vi "Read Output.vi"(8 "error in":errorcluster, 10 "byte count":i32=1000, 11 "GOLPI ref. in":T1={"pipe handle"={"lv_proc.dll file path"=path "", "process instance handle"=[]}, "fast read timeout [ms]"=500, "fast read settle time [ms]"=10, "fast read to multiple [ms]"=1, "max elements per input line"=100, "slow read timeout [ms]"=5000, "stdin double format specifier"="%_16e", "max elements per stdout output column"=100}) -> (0 "error out":errorcluster, 2 "read buffer":string, 3 "GOLPI ref. out":T1={"pipe handle"={"lv_proc.dll file path"=path "", "process instance handle"=[]}, "fast read timeout [ms]"=500, "fast read settle time [ms]"=10, "fast read to multiple [ms]"=1, "max elements per input line"=100, "slow read timeout [ms]"=5000, "stdin double format specifier"="%_16e", "max elements per stdout output column"=100}, 5 "bytes remaining":i32)   [LabVIEW 2013, in "GOLPI library.lvlib"]
doc: "Reads output of GNU Octave buffered in stdout pipe. Returns number of bytes remaining in the stdout (if any)."
uses:
  GOLPI library.lvlib
  Private/Type Definitions/GOLPI reference Type Def.ctl
  LV Process source distribution/Pipe Handle.ctl
  LV Process source distribution/LV Process library.lvlib
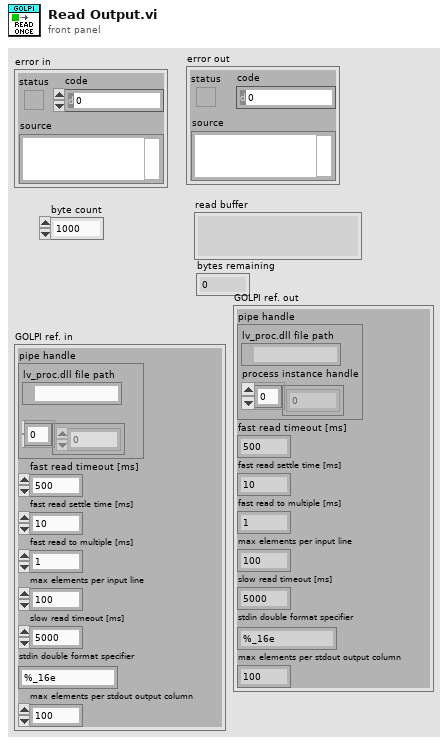
[diagram p1: front panel]
types:
  T1 = typedef "GOLPI library.lvlib/GOLPI reference Type Def.ctl" = cluster{"pipe handle":T2, "fast read timeout [ms]":u32, "fast read settle time [ms]":u32, "fast read to multiple [ms]":u32, "max elements per input line":u32, "slow read timeout [ms]":u32, "stdin double format specifier":string, "max elements per stdout output column":u32}
  T2 = typedef "LV Process library.lvlib/Pipe Handle.ctl" = cluster{"lv_proc.dll file path":path, "process instance handle":u32[]}
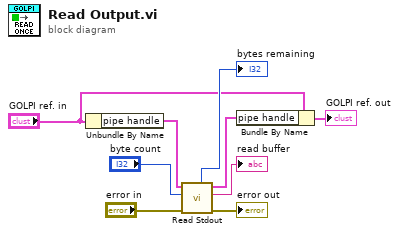
[diagram p0: block diagram]
diagram:
  n1 = Unbundle By Name("GOLPI ref. in") -> ("pipe handle"=w2:T2)
  n2 = call "Read Stdout.vi"("error in"="error in", "byte count"="byte count", "pipe in"=w2) -> ("error out"=→"error out":errorcluster, "read buffer"=→"read buffer":string, "pipe out"=w1:T2, "bytes remaining"=→"bytes remaining":i32)  [unwired: 3 in, 2 out]
  n3 = Bundle By Name(cluster="GOLPI ref. in", "pipe handle"=w1) -> (→"GOLPI ref. out":T1)
